vi "FolderToJson.vi"(8 "error in":errorcluster, 11 "Source":path) -> (0 "error out":errorcluster, 2 "Paths out":T1[](array[typedef]), 3 "resulting string":string)   [LabVIEW 2017]
uses:
  SourceJsonPaths.ctl
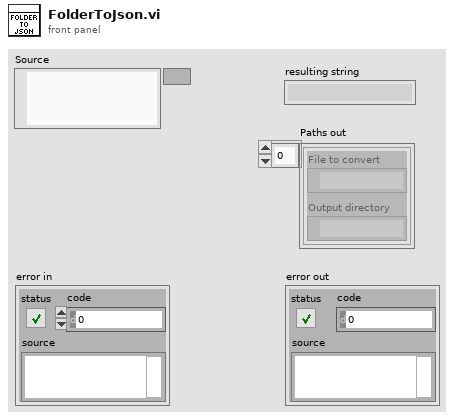
[diagram p1: front panel]
types:
  T1 = typedef "SourceJsonPaths.ctl" = cluster{"File to convert":path, "Output directory":path}
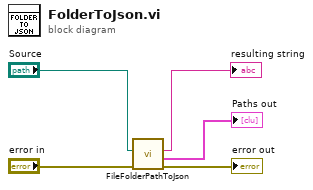
[diagram p0: block diagram]
diagram:
  n1 = call "FileFolderPathToJson.vi"("error in (no error)"="error in", "Path"="Source") -> ("error out"=→"error out":errorcluster, "Paths out"=→"Paths out":T1[], "String"=→"resulting string":string)  [unwired: 6 in, 1 out]
